vi "Get Sciscan Scope Focus.vi"(8 "error in":errorcluster, 11 "GFG Refnum":refnum<vi>) -> (0 "error out":errorcluster, 2 "Focus Status":bool, 3 "GFG Refnum Out":refnum<vi>)   [LabVIEW 2012, in "Sciscan Scope Daemon.lvlib"]
uses:
  Sciscan Scope Daemon.lvlib
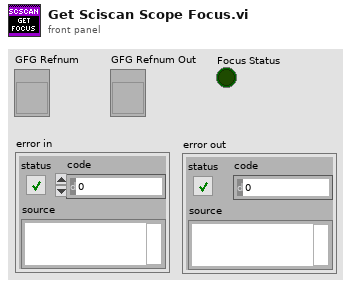
[diagram p1: front panel]
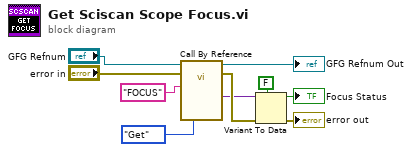
[diagram p0: block diagram]
diagram:
  n1 = call-by-ref "?"(reference="GFG Refnum", error in="error in", "Variable Name in"="FOCUS", "Action"=enum16{"Init", "Set", "Get"}."Get") -> (reference out=→"GFG Refnum Out":refnum<vi>, error out=w7:errorcluster, "Variant Out"=w6:variant)  [unwired: 11 in, 6 out]
  n2 = Variant To Data(error in=w7, type=FALSE, Variant=w6) -> (data=→"Focus Status":bool, error out=→"error out":errorcluster)
